vi "extract core.vi"(4 "Y offset":i32, 6 "X offset":i32, 7 "Region":T1(ring), 10 "Core extraction size":i32, 11 "I/P array":i16[][](array[numeric])) -> (3 "O/P array":i16[][](array[numeric]))   [LabVIEW 2020]
panel:
  in  "Intensity Graph colour palette":cluster{dbl, "Color Box":u32}[](array[cluster])=[{1000.0, "Color Box"=16714752}, {750.0, "Color Box"=15859456}, {500.0, "Color Box"=65289}, {250.0, "Color Box"=983260}, {0.0, "Color Box"=14418124}]
  out "Intensity Graph 3":i16[][](graph)
  out "dim2_length":i32
  out "dim2_start":i32
  out "dim1_length":i32
  out "dim1_start":i32
  out "output variable 6":dbl
  out "output variable 5":dbl
  out "output variable 4":dbl
  out "output variable 3":dbl
  out "output variable 2":i32
  out "output variable":i32
  out "size(s)":i32[](array[numeric])
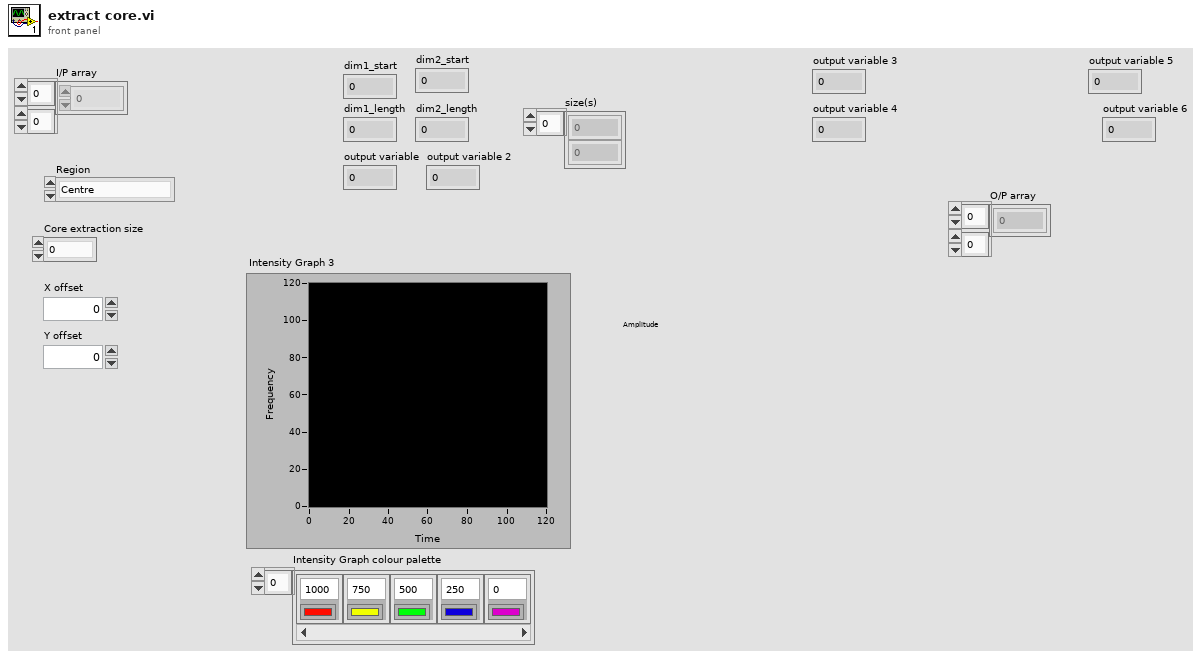
[diagram p1: front panel]
types:
  T1 = enum16{"Centre", "Top Right", "Top left", "Bottom Right", "Bottom Left"}
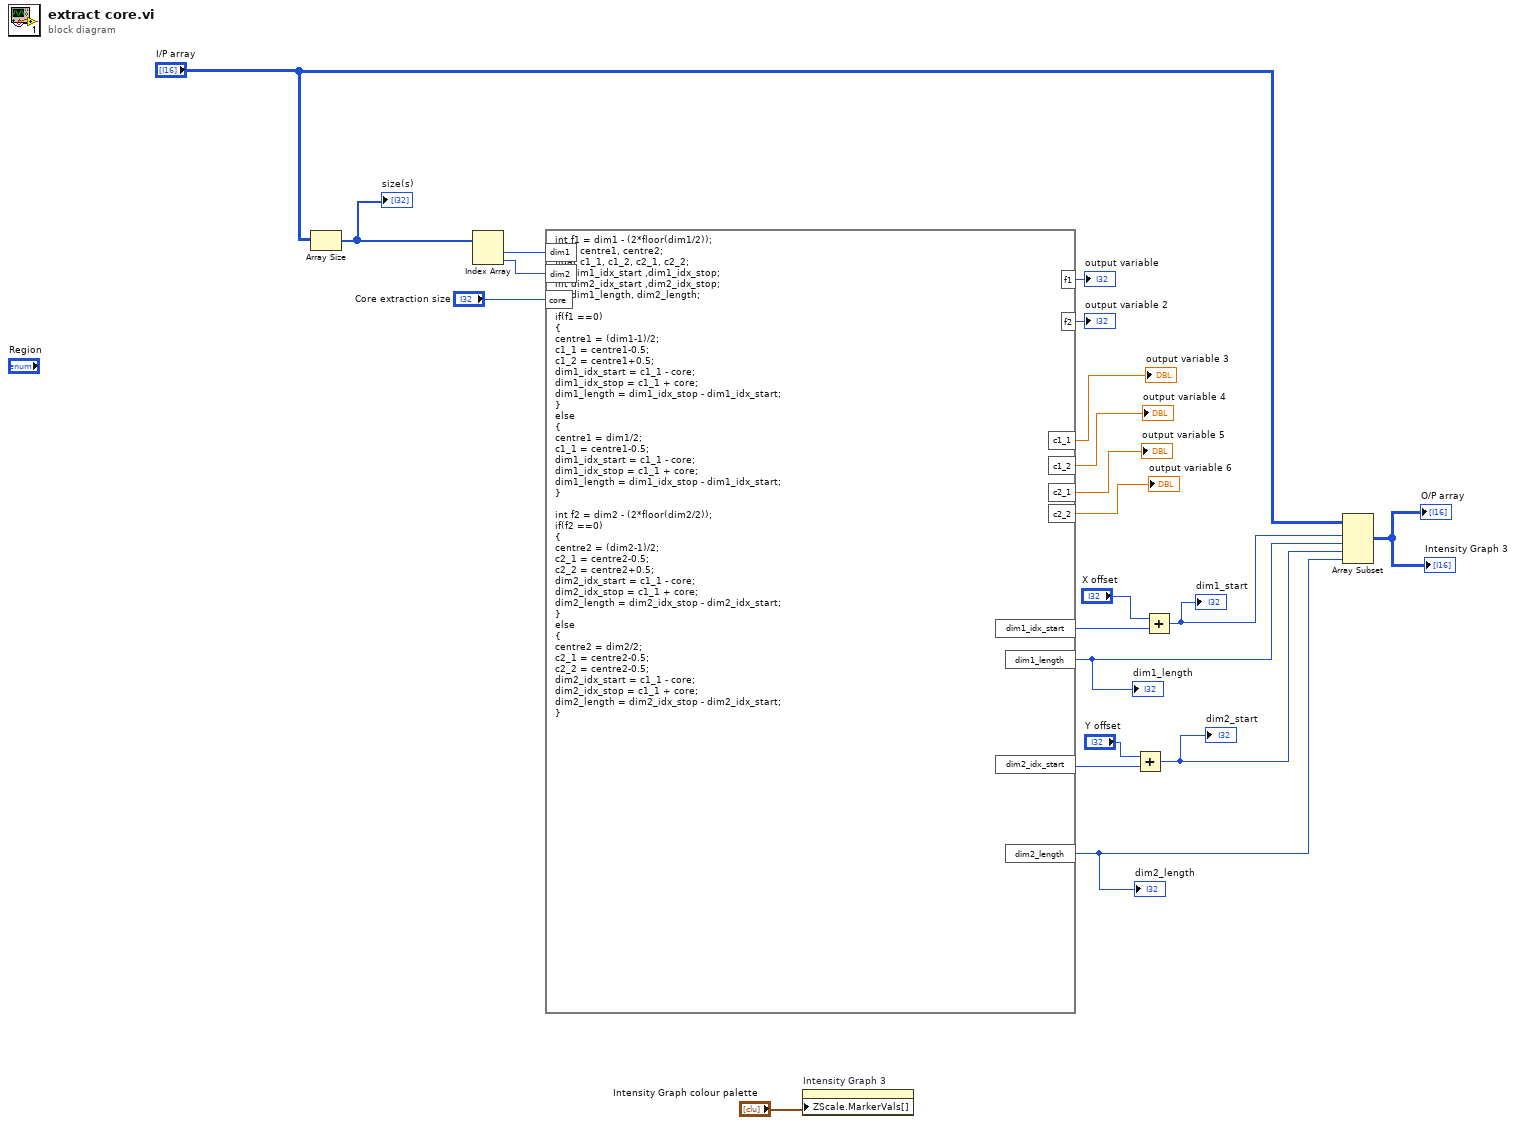
[diagram p0: block diagram]
diagram:
  n1 = Array Size(array="I/P array") -> (size(s)=w21:i32[])
  "size(s)" <- w21
  n2 = Index Array(array=w21) -> (element #1=w20:i32, element #2=w19:i32)  [unwired: 2 in]
  n3 = formula code="int f1 = dim1 - (2*floor(dim1/2));\nfloat centre1, centre2;\nfloat c1_1, c1_2, c2_1, c2_2;\nint dim1_idx_start ,dim1_idx_stop;\nint dim2_idx_start ,dim2_idx_stop;\nint dim1_length, dim2_length;\n\nif(f1 ==0)\n{\ncentre1 = (dim1-1)/2;\nc1_1 = centre1-0.5;\nc1_2 = centre1+0.5;\ndim1_idx_start = c1_1 - core;\ndim1_idx_stop = c1_1 + core;\ndim1_length = dim1_idx_stop - dim1_idx_start;\n}\nelse\n{\ncentre1 = dim1/2;\nc1_1 = centre1-0.5;\ndim1_idx_start = c1_1 - core;\ndim1_idx_stop = c1_1 + core;\ndim1_length = dim1_idx_stop - dim1_idx_start;\n}\n\nint f2 = dim2 - (2*floor(dim2/2));\nif(f2 ==0)\n{\ncentre2 = (dim2-1)/2;\nc2_1 = centre2-0.5;\nc2_2 = centre2+0.5;\ndim2_idx_start = c1_1 - core;\ndim2_idx_stop = c1_1 + core;\ndim2_length = dim2_idx_stop - dim2_idx_start;\n}\nelse\n{\ncentre2 = dim2/2;\nc2_1 = centre2-0.5; \nc2_2 = centre2-0.5;\ndim2_idx_start = c1_1 - core;\ndim2_idx_stop = c1_1 + core;\ndim2_length = dim2_idx_stop - dim2_idx_start;\n}"("dim1"=w20, "dim2"=w19, "core"="Core extraction size") -> ("f1"=→"output variable":i32, "f2"=→"output variable 2":i32, "c1_1"=→"output variable 3":dbl, "c1_2"=→"output variable 4":dbl, "c2_1"=→"output variable 5":dbl, "c2_2"=→"output variable 6":dbl, "dim1_idx_start"=w6:i32, "dim1_length"=w11:i32, "dim2_idx_start"=w3:i32, "dim2_length"=w7:i32)
  "dim1_length" <- w11
  "dim2_length" <- w7
  n4 = property on="Intensity Graph 3" class="IntGraph (strict)"("ZScale.MarkerVals[]"="Intensity Graph colour palette") -> ()  [unwired: 2 in, 2 out]
  n5 = Add(x="Y offset", y=w3) -> (x+y=w2:i32)
  "dim2_start" <- w2
  n6 = Add(x="X offset", y=w6) -> (x+y=w4:i32)
  "dim1_start" <- w4
  n7 = Array Subset(array="I/P array", index (row)=w4, length (row)=w11, index (col)=w2, length (col)=w7) -> (→"Intensity Graph 3" →"O/P array":i16[][])
